vi "lab_1.vi"() -> ()   [LabVIEW 2022 SP3]
panel:
  out "R=X-Y":dbl
  out "Z=X+Y":dbl
  in  "Y":dbl
  in  "X":dbl
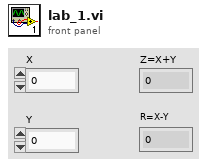
[diagram p1: front panel]
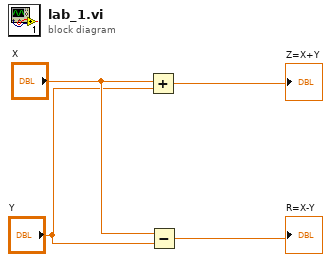
[diagram p0: block diagram]
diagram:
  n1 = Add(x="X", y="Y") -> (x+y=→"Z=X+Y":dbl)
  n2 = Subtract(x="X", y="Y") -> (x-y=→"R=X-Y":dbl)
